vi "Get Joystick.vi"() -> (6 "Joystick Controls":T1)   [LabVIEW 2017]
uses:
  Joystick Controls.ctl
  Refnum Names.vi
  <vilib>/Rock Robotics/WPI/Utilities/WPI_GetSetVariantRefNum.vi
panel:
  in  "Joystick Controls":T1
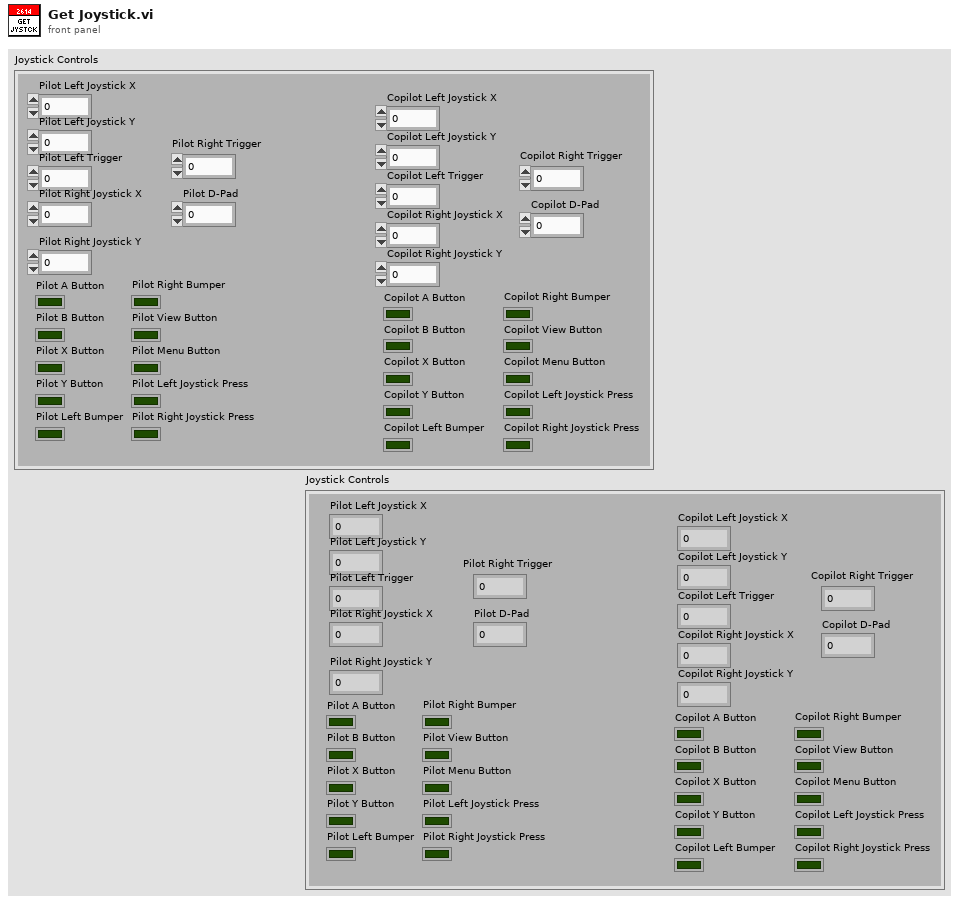
[diagram p1: front panel]
types:
  T1 = typedef "Joystick Controls.ctl" = cluster{"Pilot Left Joystick X":dbl, "Pilot Left Joystick Y":dbl, "Pilot A Button":bool, "Pilot B Button":bool, "Pilot X Button":bool, "Pilot Y Button":bool, "Pilot Left Bumper":bool, "Pilot Right Bumper":bool, "Pilot View Button":bool, "Pilot Menu Button":bool, "Pilot Left Joystick Press":bool, "Pilot Right Joystick Press":bool, "Pilot Left Trigger":dbl, "Pilot Right Joystick X":dbl, "Pilot Right Joystick Y":dbl, "Pilot Right Trigger":dbl, "Copilot Left Joystick X":dbl, "Copilot Left Joystick Y":dbl, "Copilot A Button":bool, "Copilot B Button":bool, "Copilot X Button":bool, "Copilot Y Button":bool, "Copilot Left Bumper":bool, "Copilot Right Bumper":bool, "Copilot View Button":bool, "Copilot Menu Button":bool, "Copilot Left Joystick Press":bool, "Copilot Right Joystick Press":bool, "Copilot Left Trigger":dbl, "Copilot Right Joystick X":dbl, "Copilot Right Joystick Y":dbl, "Copilot Right Trigger":dbl, "Pilot D-Pad":i16, "Copilot D-Pad":i16}
  T2 = typedef "WPI_JoystickDevRef.ctl" = cluster{"Device":T3}
  T3 = typedef "WPI_JoystickDeviceEnum.ctl" = enum16{"USB 0", "USB 1", "USB 2", "USB 3", "USB 4", "USB 5"}
  T4 = cluster{"Axes[0]":dbl, "Axes[1]":dbl, "Axes[2]":dbl, "Axes[3]":dbl, "Axes[4]":dbl, "Axes[5]":dbl, "Axes[6]":dbl, "Axes[7]":dbl, "Axes[8]":dbl}
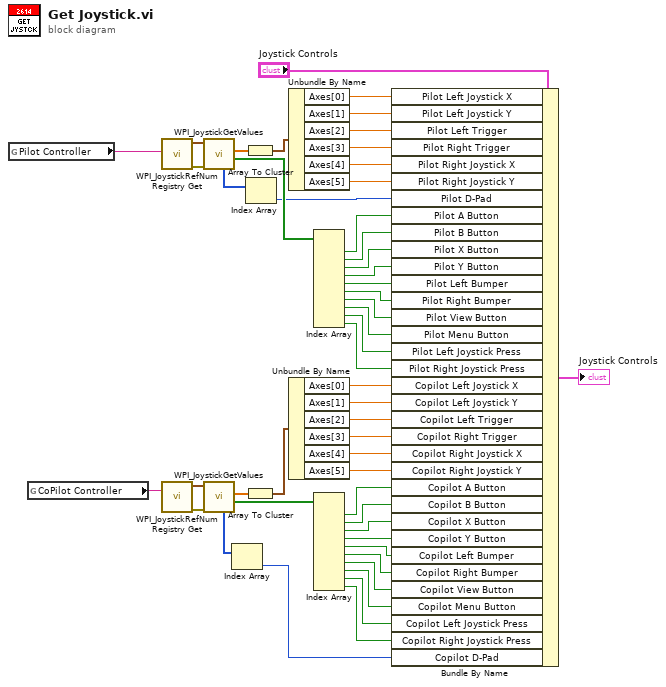
[diagram p0: block diagram]
diagram:
  n1 = global read "Refnum Names.vi" "Pilot Controller"() -> (w6:string)
  n2 = global read "Refnum Names.vi" "CoPilot Controller"() -> (w5:string)
  n3 = call <vilib>:"WPI_JoystickRefNum Registry Get.vi"("refnum name"=w6) -> ("error out"=w2:errorcluster, "JoystickDevRef"=w50:T2)  [unwired: 9 in]
  n4 = call <vilib>:"WPI_JoystickRefNum Registry Get.vi"("refnum name"=w5) -> ("error out"=w1:errorcluster, "JoystickDevRef"=w30:T2)  [unwired: 9 in]
  n5 = call <vilib>:"WPI_JoystickGetValues.vi"("error in (no error)"=w2, "JoystickDevRef"=w50) -> ("Buttons"=w41:bool[], "Axes"=w49:dbl[], "POVs"=w8:i16[])  [unwired: 5 in, 2 out]
  n6 = call <vilib>:"WPI_JoystickGetValues.vi"("error in (no error)"=w1, "JoystickDevRef"=w30) -> ("Buttons"=w28:bool[], "Axes"=w29:dbl[], "POVs"=w4:i16[])  [unwired: 5 in, 2 out]
  n7 = Index Array(array=w4) -> (element=w3:i16)  [unwired: 1 in]
  n8 = Array To Cluster(array=w49) -> (cluster=w48:T4)
  n9 = Array To Cluster(array=w29) -> (cluster=w27:T4)
  n10 = Index Array(array=w8) -> (element=w7:i16)  [unwired: 1 in]
  n11 = Unbundle By Name(w48) -> ("Axes[0]"=w47:dbl, "Axes[1]"=w46:dbl, "Axes[2]"=w45:dbl, "Axes[3]"=w44:dbl, "Axes[4]"=w43:dbl, "Axes[5]"=w42:dbl)
  n12 = Unbundle By Name(w27) -> ("Axes[0]"=w26:dbl, "Axes[1]"=w25:dbl, "Axes[2]"=w24:dbl, "Axes[3]"=w23:dbl, "Axes[4]"=w22:dbl, "Axes[5]"=w21:dbl)
  n13 = Index Array(array=w41) -> (element #1=w40:bool, element #2=w39:bool, element #3=w38:bool, element #4=w37:bool, element #5=w36:bool, element #6=w35:bool, element #7=w34:bool, element #8=w33:bool, element #9=w32:bool, element #10=w31:bool)  [unwired: 10 in]
  n14 = Index Array(array=w28) -> (element #1=w20:bool, element #2=w19:bool, element #3=w18:bool, element #4=w17:bool, element #5=w15:bool, element #6=w16:bool, element #7=w14:bool, element #8=w13:bool, element #9=w12:bool, element #10=w11:bool)  [unwired: 10 in]
  n15 = Bundle By Name(cluster="Joystick Controls", "Pilot Left Joystick X"=w47, "Pilot Left Joystick Y"=w46, "Pilot Left Trigger"=w45, "Pilot Right Trigger"=w44, "Pilot Right Joystick X"=w43, "Pilot Right Joystick Y"=w42, "Pilot D-Pad"=w7, "Pilot A Button"=w40, "Pilot B Button"=w39, "Pilot X Button"=w38, "Pilot Y Button"=w37, "Pilot Left Bumper"=w36, "Pilot Right Bumper"=w35, "Pilot View Button"=w34, "Pilot Menu Button"=w33, "Pilot Left Joystick Press"=w32, "Pilot Right Joystick Press"=w31, "Copilot Left Joystick X"=w26, "Copilot Left Joystick Y"=w25, "Copilot Left Trigger"=w24, "Copilot Right Trigger"=w23, "Copilot Right Joystick X"=w22, "Copilot Right Joystick Y"=w21, "Copilot A Button"=w20, "Copilot B Button"=w19, "Copilot X Button"=w18, "Copilot Y Button"=w17, "Copilot Left Bumper"=w15, "Copilot Right Bumper"=w16, "Copilot View Button"=w14, "Copilot Menu Button"=w13, "Copilot Left Joystick Press"=w12, "Copilot Right Joystick Press"=w11, "Copilot D-Pad"=w3) -> (→"Joystick Controls":T1)
